vi "Set Home (SubVI).vi"(7 "Home Offset (deg)":dbl, 8 "error in (no error)":errorcluster, 11 "VISA Refnum in":refnum<visa-resource-name>) -> (0 "error out":errorcluster, 3 "VISA Refnum out":refnum<visa-resource-name>)   [LabVIEW 2012]
uses:
  <instrlib>/ZaberTSeries/Public/Utility/Request.ctl
  <instrlib>/ZaberTSeries/ZaberTSeries.lvlib
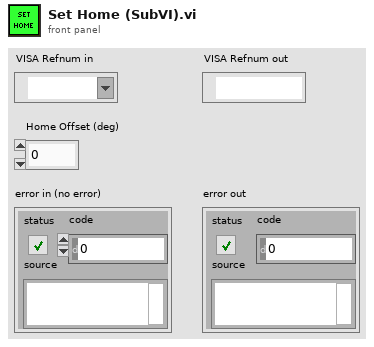
[diagram p1: front panel]
types:
  T1 = typedef "ZaberTSeries.lvlib/Request.ctl" = cluster{"Device Number":u8, "Command":u8, "Data":i32, "Response Count":i32}
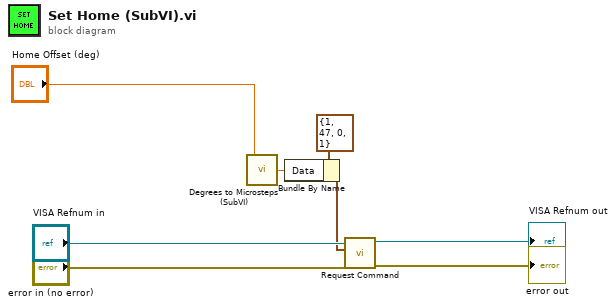
[diagram p0: block diagram]
diagram:
  n1 = call "Degrees to Microsteps (SubVI).vi"("Degrees"="Home Offset (deg)") -> ("Microsteps"=w1:dbl)  [unwired: 4 in]
  n2 = Bundle By Name(cluster=T1 {"Device Number"=1, "Command"=47, "Data"=0, "Response Count"=1} ("Request"), "Data"=w1) -> (w4:T1)
  n3 = call <instrlib>:"Request Command.vi"("error in (no error)"="error in (no error)", "Request"=w4, "VISA resource name"="VISA Refnum in") -> ("error out"=→"error out":errorcluster, "VISA resource name out"=→"VISA Refnum out":refnum<visa-resource-name>)  [unwired: 5 in, 2 out]
